vi "Read Path in.vi"(8 "error in (no error)":errorcluster, 11 "[Test Case] Fix Path in":refnum<class "[Test Case] Fix path.lvclass">) -> (0 "error out":errorcluster, 2 "Path in":string, 3 "[Test Case] Fix Path out":refnum<class "[Test Case] Fix path.lvclass">)   [LabVIEW 2015, in "Tests.lvlib" / "[Test Case] Fix path.lvclass"]
uses:
  [Test Case] Fix path.lvclass
  [Test Case] Fix path.lvclass/[Test Case] Fix path.ctl
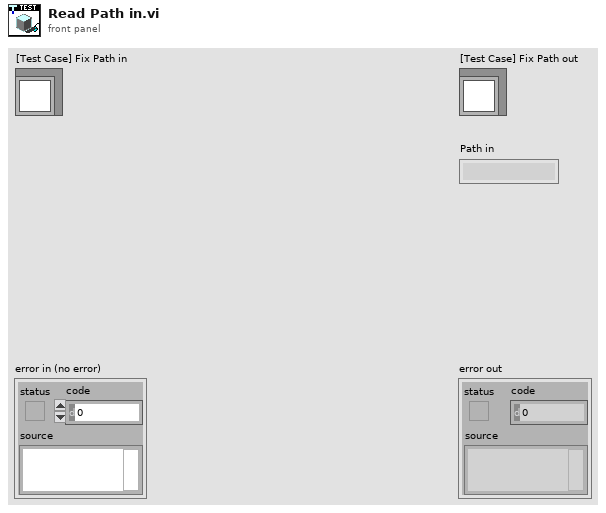
[diagram p1: front panel]
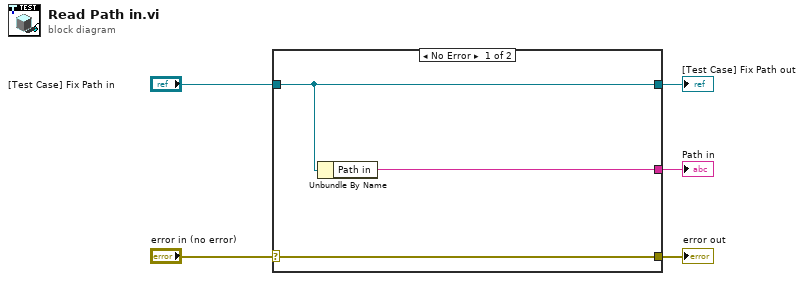
[diagram p0: block diagram]
diagram:
  n1 = case shown="No Error" "error in (no error)" {
    selector: "error in (no error)" -> [w8 w9]
    tunnel: [w8 w9] -> w4
    tunnel: [w7 w10] -> w2
    tunnel: "[Test Case] Fix Path in" -> [w7 w10]
    tunnel: [w6 _] -> w1
    frame No Error {
      n2 = Unbundle By Name(w7) -> ("Path in"=w6:string)
    }
    frame Error {
    }
  }
  "error out" <- w4
  "[Test Case] Fix Path out" <- w2
  "Path in" <- w1
